vi "PushOpen.vi"(10 "node ref in":refnum<data-value>, 11 "RVCLibrary_Bug in":refnum<class "RVCLibrary_Bug2.lvclass">) -> (2 "node ref out":refnum<data-value>, 3 "RVCLibrary_Bug out":refnum<class "RVCLibrary_Bug2.lvclass">)   [LabVIEW 2013, in "RVCLibrary_Bug2.lvclass"]
uses:
  RVCLibrary_Bug2.lvclass
  <vilib>/robotics/Navigation/shared/MapNode/AbstractDstarNode/NI_Robotics_AbstractDstarNode.lvclass
  RVCLibrary_Bug2.lvclass/RVCLibrary_Bug2.ctl
  <vilib>/robotics/Navigation/shared/Priority Queue/Open List Element.ctl
  <vilib>/robotics/Navigation/shared/MapNode/AbstractMapNode/NI_Robotics_AbstractMapNode.lvclass
  <vilib>/robotics/Navigation/shared/Priority Queue/NI_Robotics_Priority Queue.lvclass
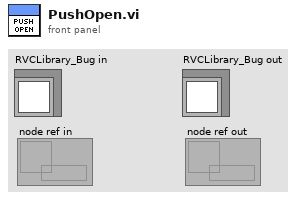
[diagram p1: front panel]
types:
  T1 = typedef "NI_Robotics_Priority Queue.lvclass/Open List Element.ctl" = cluster{"f":dbl, "g":dbl, "node Ref":refnum<data-value>}
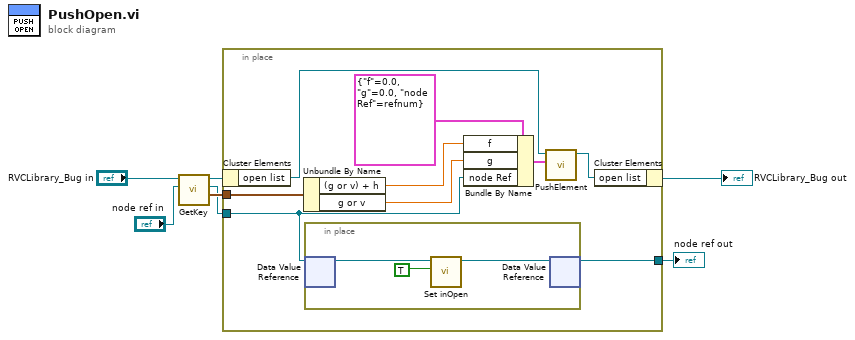
[diagram p0: block diagram]
diagram:
  n1 = call "GetKey.vi"("node ref in"="node ref in", "RVCLibrary_Bug2 in"="RVCLibrary_Bug in") -> ("key out"=w6:cluster{"(g or v) + h":dbl, "g or v":dbl}, "node ref out"=w4:refnum<data-value>, "RVCLibrary_Bug2 out"=w7:refnum<class "RVCLibrary_Bug2.lvclass">)  [unwired: 7 in]
  n2 = in-place {
    in-place-border: w6 -> [w12]
    in-place-border: w4 -> [w9]
    in-place-border: [w8] -> w3
    n3 = in-place-cluster #1(w7) -> ("open list"=w14:refnum<class "NI_Robotics_Priority Queue.lvclass">)
    n4 = Unbundle By Name(w12) -> ("(g or v) + h"=w11:dbl, "g or v"=w10:dbl)
    n5 = in-place {
      n6 = in-place-dvr #2(w9) -> (w18:refnum<class "NI_Robotics_AbstractDstarNode.lvclass">)  [unwired: 1 out]
      n7 = call <vilib>:"Set inOpen.vi"("inOpen"=TRUE, "AbstractDstarNode in"=w18) -> ("AbstractDstarNode out"=w17:refnum<class "NI_Robotics_AbstractDstarNode.lvclass">)  [unwired: 8 in, 1 out]
      n8 = in-place-dvr #2(w17) -> (w8:refnum<data-value>)  [unwired: 1 out]
    }
    n9 = Bundle By Name(cluster=T1 {"f"=0.0, "g"=0.0, "node Ref"=refnum} ("Open List Element"), "f"=w11, "g"=w10, "node Ref"=w9) -> (w16:T1)
    n10 = call <vilib>:"PushElement.vi"("open list element"=w16, "Astar Open List in"=w14) -> ("Astar Open List out"=w13:refnum<class "NI_Robotics_Priority Queue.lvclass">)  [unwired: 8 in, 1 out]
    n11 = in-place-cluster #1("open list"=w13) -> (→"RVCLibrary_Bug out":refnum<class "RVCLibrary_Bug2.lvclass">)
  }
  "node ref out" <- w3
